vi "NaN Points out of Domain and Range.vi"(10 "Data in":dbl[](array[numeric]), 11 "Exponential Fit in":refnum<class "Exponential Fit.lvclass">) -> (2 "Data out":dbl[](array[numeric]), 3 "Exponential Fit out":refnum<class "Exponential Fit.lvclass">)   [LabVIEW 2016, in "Exponential Fit.lvclass"]
uses:
  Exponential Fit.lvclass
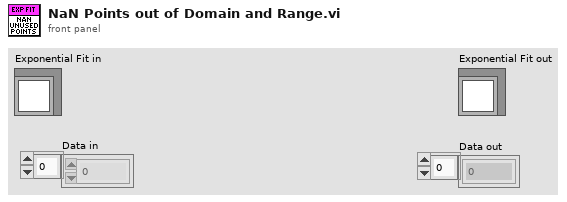
[diagram p1: front panel]
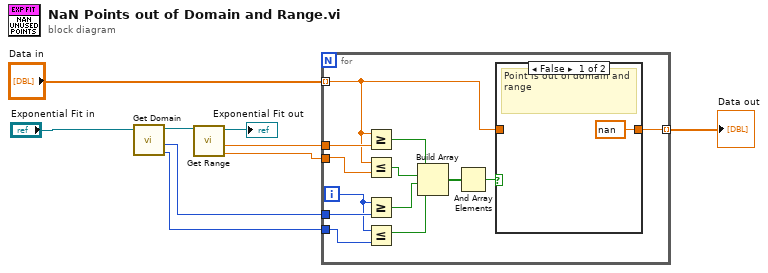
[diagram p0: block diagram]
diagram:
  n1 = call "Get Domain.vi"("Exponential Fit in"="Exponential Fit in") -> ("Xmax"=w6:i32, "Xmin"=w7:i32, "Exponential Fit out"=w8:refnum<class "Exponential Fit.lvclass">)  [unwired: 7 in, 1 out]
  n2 = call "Get Range.vi"("Exponential Fit in"=w8) -> ("Ymax"=w3:dbl, "Ymin"=w4:dbl, "Exponential Fit out"=→"Exponential Fit out":refnum<class "Exponential Fit.lvclass">)  [unwired: 7 in, 1 out]
  n3 = for {
    tunnel: "Data in" -> [w11] mode=indexing
    tunnel: w7 -> [w20]
    tunnel: w6 -> [w18]
    tunnel: w4 -> [w22]
    tunnel: w3 -> [w21]
    tunnel: [w10] -> w2 mode=indexing
    i -> [w19]
    n4 = Greater Or Equal?(x=w11, y=w22) -> (x >= y?=w15:bool)
    n5 = Less Or Equal?(x=w11, y=w21) -> (x <= y?=w17:bool)
    n6 = Greater Or Equal?(x=w19, y=w20) -> (x >= y?=w13:bool)
    n7 = Less Or Equal?(x=w19, y=w18) -> (x <= y?=w14:bool)
    n8 = Build Array(w15, w17, w13, w14) -> (w16:bool[])
    n9 = And Array Elements(Boolean array=w16) -> (logical AND=w12:bool)
    n10 = case shown="False" w12 {
      tunnel: w11 -> [_ w24]
      tunnel: [nan w24] -> w10
      frame False {
        # "Point is out of domain and range"
      }
      frame True {
        # "Point is in domain and range"
      }
    }
  }
  "Data out" <- w2
